vi "Read Encoder A Channel.vi"(8 "error in (no error)":errorcluster, 11 "DriveMotors in":refnum<class "DriveMotors.lvclass">) -> (0 "error out":errorcluster, 2 "DIOChannel":T1, 3 "DriveMotors out":refnum<class "DriveMotors.lvclass">)   [LabVIEW 2013, in "DriveMotors.lvclass"]
uses:
  DriveMotors.lvclass
  <vilib>/Rock Robotics/SystemInterfaces/DIO/FPGA_DIOChannel.ctl
  DriveMotors.lvclass/DriveMotors.ctl
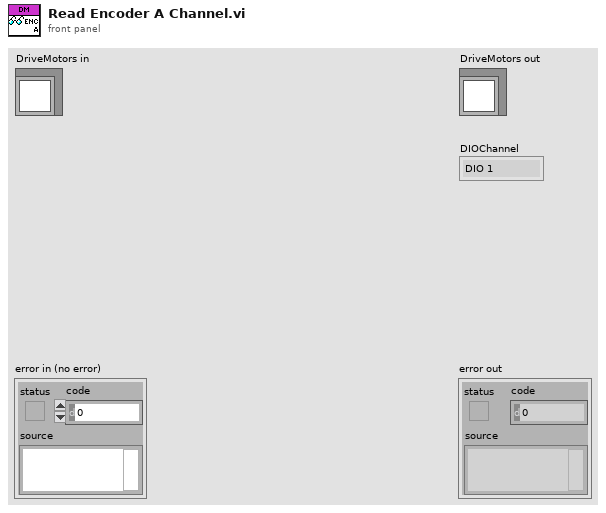
[diagram p1: front panel]
types:
  T1 = typedef "FPGA_DIOChannel.ctl" = enum8{"DIO 1", "DIO 2", "DIO 3", "DIO 4", "DIO 5", "DIO 6", "DIO 7", "DIO 8", "DIO 9", "DIO 10", "DIO 11", "DIO 12", "DIO 13", "DIO 14", "Invalid"}
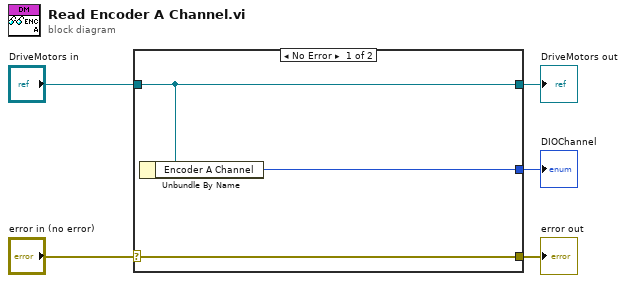
[diagram p0: block diagram]
diagram:
  n1 = case shown="No Error" "error in (no error)" {
    selector: "error in (no error)" -> [w8 w9]
    tunnel: [w8 w9] -> w4
    tunnel: [w7 w10] -> w2
    tunnel: "DriveMotors in" -> [w7 w10]
    tunnel: [w6 _] -> w1
    frame No Error {
      n2 = Unbundle By Name(w7) -> ("Encoder A Channel"=w6:T1)
    }
    frame Error {
    }
  }
  "error out" <- w4
  "DriveMotors out" <- w2
  "DIOChannel" <- w1
